vi "Fetch Waveform Measurement (Communication).vi"(0 "VISA resource name":refnum<visa-resource-name>, 5 "Channel (0:Channel1)":u16(ring) items=["Channel 1", "Channel 2", "Channel 3", "Channel 4", "Math 1", "Math 2", "Math 3", "Math 4", "Reference 1", "Reference 2", "Reference 3", "Reference 4"], 7 "Function (0:Ext Ratio)":u16(ring) items=["Ext Ratio", "Ext Ratio%", "Ext Ratio (dB)", "Eye Height", "Eye Top", "Eye Width", "Eye Base", "Crossing%", "Jitter P-P", "Noise P-P", "Cyc Distortion", "Jitter RMS", "Noise RMS", "Q-Factor", "Jitter 6", "S/N Ratio"], 11 "error in (no error)":errorcluster) -> (4 "VISA resource name out":refnum<visa-resource-name>, 6 "Measurement":dbl, 15 "error out":errorcluster)   [LabVIEW 2015, in "Tektronix 7000 Series.lvlib"]
doc: "Initiates a waveform acquisition on the specified <B>Channel</B> and returns a <B>Measurement</B> value. Use the Fetch Waveform Measurement VI separately for any other waveform measurement on a channel without initiating another acquisition."
uses:
  <instrlib>/Tektronix 7000 Series/Tektronix 7000 Series.lvlib
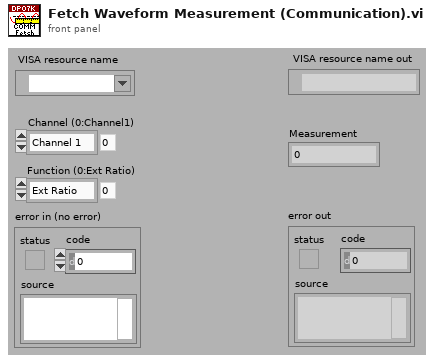
[diagram p1: front panel]
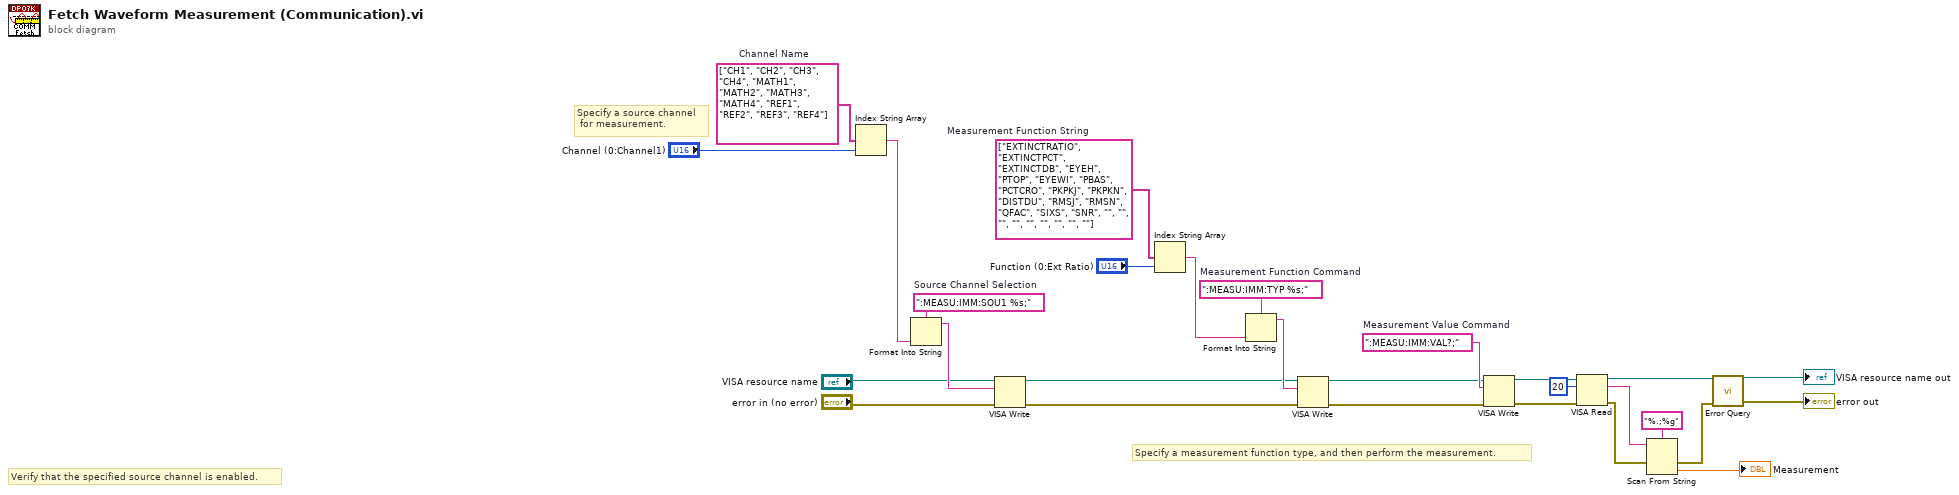
[diagram p0: block diagram]
diagram:
  w9 = string[] ["CH1", "CH2", "CH3", "CH4", "MATH1", "MATH2", "MATH3", "MATH4", "REF1", "REF2", "REF3", "REF4"]  # Channel Name
  w14 = ":MEASU:IMM:SOU1 %s;"  # Source Channel Selection
  w24 = ":MEASU:IMM:VAL?;"  # Measurement Value Command
  w27 = ":MEASU:IMM:TYP %s;"  # Measurement Function Command
  w28 = string[] ["EXTINCTRATIO", "EXTINCTPCT", "EXTINCTDB", "EYEH", "PTOP", "EYEWI", "PBAS", "PCTCRO", "PKPKJ", "PKPKN", "DISTDU", "RMSJ", "RMSN", "QFAC", "SIXS", "SNR", "", "", "", "", "", "", "", "", ""]  # Measurement Function String
  # "Specify a measurement function type, and then perform the measurement."
  # "Specify a source channel\n for measurement."
  # "Verify that the specified source channel is enabled."
  n1 = Index String Array(1:"Channel (0:Channel1)", 2:w9) -> (0:w15:string)  [unwired: 1 in]
  n2 = Format Into String(format string=w14, w15) -> (resulting string=w13:string)  [unwired: 2 in, 1 out]
  n3 = VISA Write(VISA resource name="VISA resource name", write buffer=w13, error in (no error)="error in (no error)") -> (VISA resource name out=w11:refnum<visa-resource-name>, error out=w10:errorcluster)  [unwired: 1 out]
  n4 = Index String Array(1:"Function (0:Ext Ratio)", 2:w28) -> (0:w26:string)  [unwired: 1 in]
  n5 = Format Into String(format string=w27, w26) -> (resulting string=w25:string)  [unwired: 2 in, 1 out]
  n6 = VISA Write(VISA resource name=w11, write buffer=w25, error in (no error)=w10) -> (VISA resource name out=w17:refnum<visa-resource-name>, error out=w16:errorcluster)  [unwired: 1 out]
  n7 = VISA Write(VISA resource name=w17, write buffer=w24, error in (no error)=w16) -> (VISA resource name out=w23:refnum<visa-resource-name>, error out=w22:errorcluster)  [unwired: 1 out]
  n8 = VISA Read(VISA resource name=w23, byte count=u32 20, error in (no error)=w22) -> (VISA resource name out=w5:refnum<visa-resource-name>, read buffer=w20:string, error out=w4:errorcluster)  [unwired: 1 out]
  n9 = Scan From String(format string="%.;%g", input string=w20, error in=w4) -> (error out=w3:errorcluster, output 1=→"Measurement":dbl)  [unwired: 2 in, 2 out]
  n10 = call <instrlib>:"Error Query.vi"("error in (no error)"=w3, "VISA resource name"=w5) -> ("error out"=→"error out":errorcluster, "VISA resource name out"=→"VISA resource name out":refnum<visa-resource-name>)  [unwired: 6 in, 2 out]
